vi "Time for 1.1.vi"() -> ()   [LabVIEW 2013]
panel:
  out "x-y":u32
  out "fib(n)":i32
  in  "n":i16
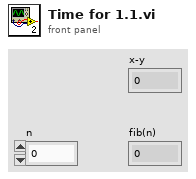
[diagram p1: front panel]
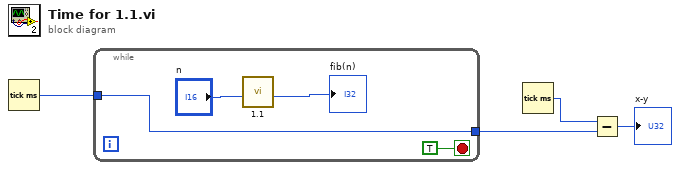
[diagram p0: block diagram]
diagram:
  n1 = Tick Count (ms)() -> (millisecond timer value=w4:u32)
  n2 = while {
    tunnel: w4 -> [w5]
    tunnel: [w5] -> w2
    stop <- TRUE stop-if-true
    n3 = call "1.1.vi"("n"="n") -> ("fib(n)"=→"fib(n)":i32)  [unwired: 10 in]
  }
  n4 = Tick Count (ms)() -> (millisecond timer value=w3:u32)
  n5 = Subtract(x=w3, y=w2) -> (x-y=→"x-y":u32)
